vi "IDS Camera Messenger.vi"(0 "Notifier Name":string, 2 "IDS Actions":T5, 5 "IDS Parameter":T1, 7 "ROI Setup":T3, 9 "# of Frames":u32, 11 "File Save Path":path) -> (4 "Notifier Name (Dup)":string, 6 "IDS Parameter":T1, 8 "IDS ROI":T3, 10 "Running?":bool, 13 "Image Ref":T4, 15 "Error?":bool)   [LabVIEW 2025]
uses:
  IDS Controls/IDS Actions.ctl
  IDS Controls/IDS Parameters.ctl
  IDS Controls/IDS Parameter List.ctl
  IDS Controls/IDS ROI.ctl
  <vilib>/vision/Image Controls.llb/IMAQ Image.ctl
  IDS Controls/IDS Notifier Element.ctl
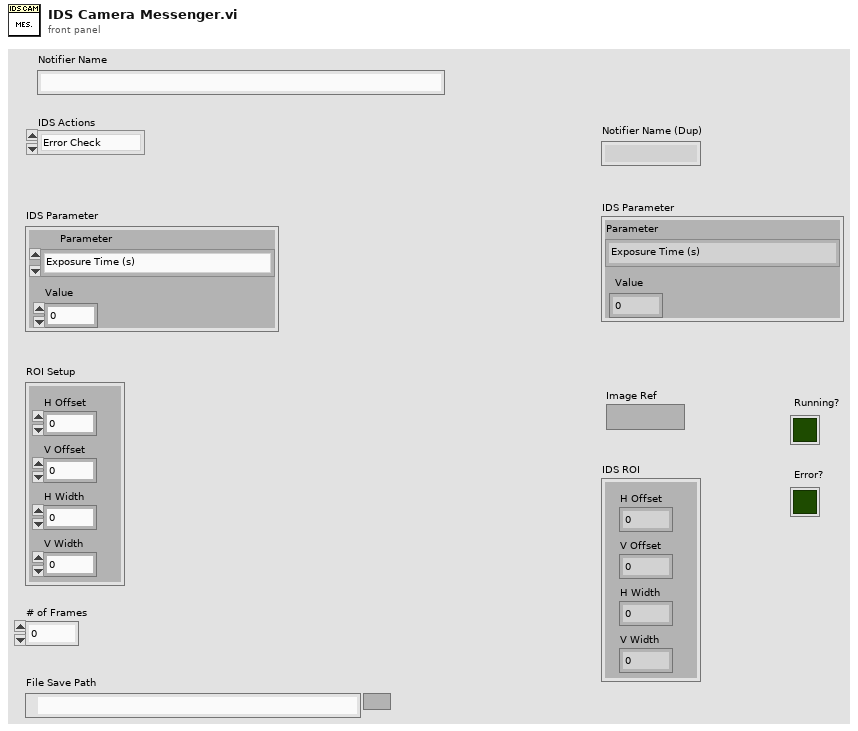
[diagram p1: front panel]
types:
  T1 = typedef "IDS Parameters.ctl" = cluster{"Parameter":T2, "Value":dbl}
  T2 = typedef "IDS Parameter List.ctl" = enum16{"Exposure Time (s)", "Binning"}
  T3 = typedef "IDS ROI.ctl" = cluster{"H Offset":i32, "V Offset":i32, "H Width":i32, "V Width":i32}
  T4 = typedef "IMAQ Image.ctl" = refnum<image>
  T5 = typedef "IDS Actions.ctl" = enum16{"Error Check", "Initialize", "Preview", "Record", "Abort", "Record Settings", "Set Parameter", "Get Parameter", "Set ROI", "Get ROI", "Status", "Quit"}
  T6 = typedef "IDS Notifier Element.ctl" = cluster{"IDS Actions":T5, "Received?":bool, "IDS Parameter":T1, "IDS ROI":T3, "Running?":bool, "File Path":path, "# of frames":u32, "Image Ref":T4, "Error":errorcluster, "Binning":i32}
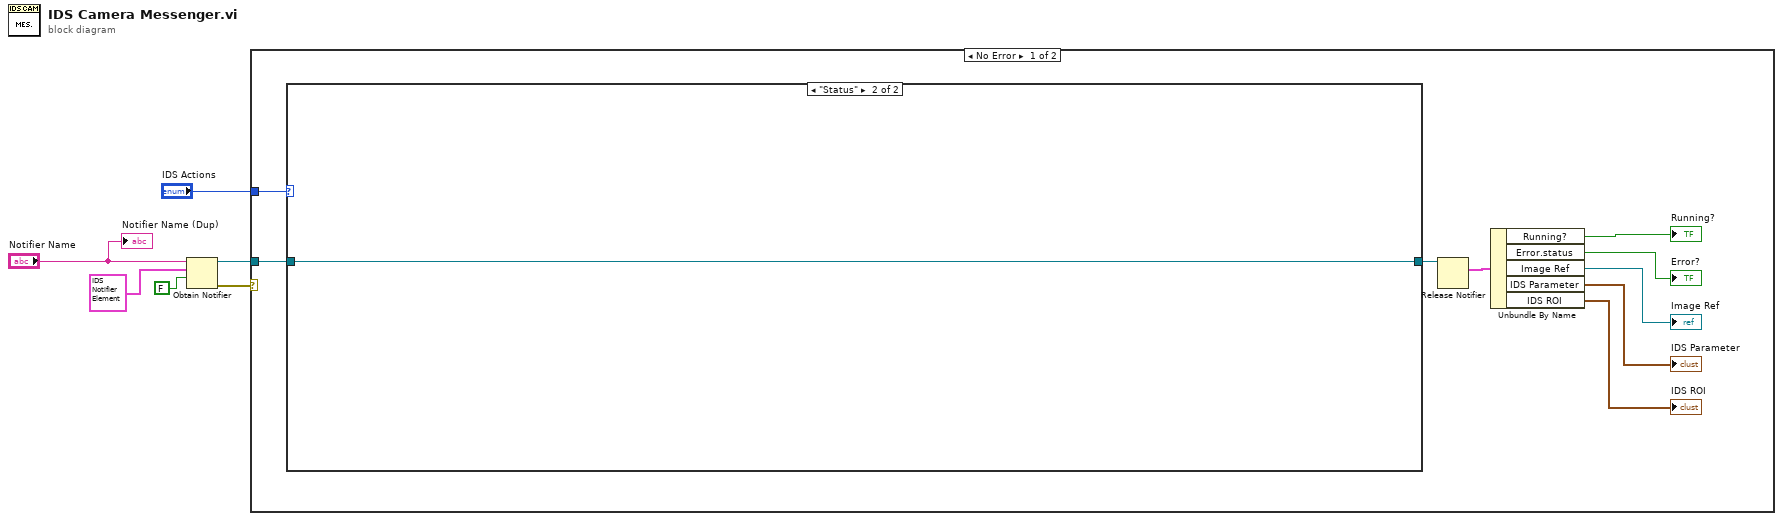
[diagram p0: block diagram]
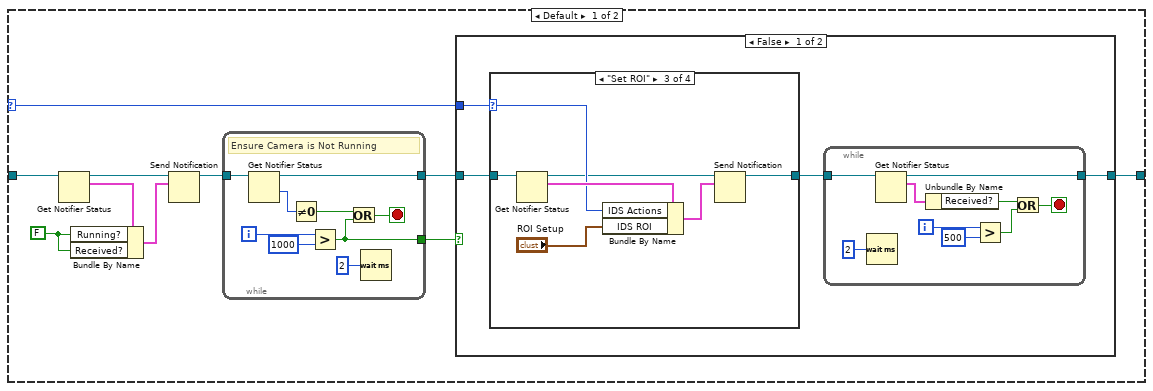
[diagram p2: hidden frame]
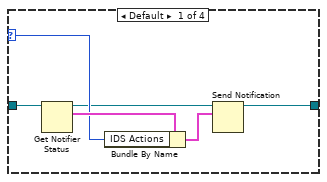
[diagram p3: hidden frame]
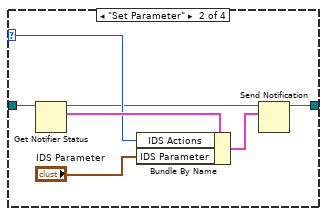
[diagram p4: hidden frame]
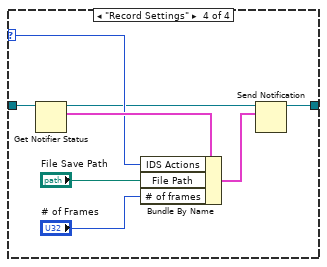
[diagram p5: hidden frame]
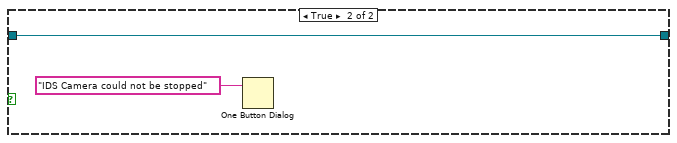
[diagram p6: hidden frame]
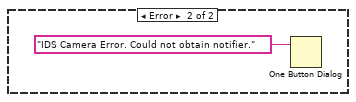
[diagram p7: hidden frame]
diagram:
  n1 = Obtain Notifier(name (unnamed)="Notifier Name", notification data type=T6 {"IDS Actions"=enum."Quit", "Received?"=TRUE, "IDS Parameter"={"Parameter"=enum."Exposure Time (s)", "Value"=0.0}, "IDS ROI"={"H Offset"=0, "V Offset"=0, "H Width"=0, "V Width"=0}, "Running?"=FALSE, "File Path"=path "", "# of frames"=0, "Image Ref"=refnum, "Error"={"status"=FALSE, "code"=0, "source"=""}, "Binning"=0} ("IDS Camera Cluster"), create if not found? (T)=FALSE) -> (notifier out=w3:refnum<notifier>, error out=w4:errorcluster)  [unwired: 1 in, 1 out]
  n2 = case shown="No Error" w4 {
    tunnel: w3 -> [w15 _]
    tunnel: "IDS Actions" -> [w14 _]
    frame No Error {
      n3 = case shown="\"Status\"" w14 {
        selector: w14 -> [w21 _]
        tunnel: w15 -> [w25 w78]
        tunnel: [w20 w78] -> w8
        frame Default {
          w16 = FALSE ("Running?")
          n4 = Get Notifier Status(notifier=w25) -> (notifier out=w19:refnum<notifier>, current notification=w18:T6)  [unwired: 1 in, 3 out]
          n5 = Bundle By Name(cluster=w18, "Running?"=w16, "Received?"=w16) -> (w17:T6)
          n6 = Send Notification(notification=w17, notifier=w19) -> (notifier out=w24:refnum<notifier>)  [unwired: 1 in, 1 out]
          n7 = while {
            tunnel: w24 -> [w77]
            tunnel: [w76] -> w22
            tunnel: [w71] -> w23
            i -> [w73]
            stop <- w75 stop-if-true
            # "Ensure Camera is Not Running"
            n8 = Get Notifier Status(notifier=w77) -> (notifier out=w76:refnum<notifier>, # waiting=w70:i32)  [unwired: 1 in, 3 out]
            n9 = Not Equal To 0?(x=w70) -> (x != 0?=w69:bool)
            n10 = Greater?(x=w73, y=1000) -> (0:w71:bool)
            n11 = Or(x=w69, y=w71) -> (x .or. y?=w75:bool)
            n12 = Wait (ms)(milliseconds to wait=u32 2) -> ()  [unwired: 1 out]
          }
          n13 = case shown="False" w23 {
            tunnel: w22 -> [w27 w67]
            tunnel: w21 -> [w29 _]
            tunnel: [w26 w67] -> w20
            frame False {
              n14 = case shown="\"Set ROI\"" w29 {
                selector: w29 -> [w42 w49 w56 w64]
                tunnel: w27 -> [w44 w51 w58 w66]
                tunnel: [w39 w46 w53 w61] -> w28
                frame Default {
                  n15 = Get Notifier Status(notifier=w44) -> (notifier out=w41:refnum<notifier>, current notification=w43:T6)  [unwired: 1 in, 3 out]
                  n16 = Bundle By Name(cluster=w43, "IDS Actions"=w42) -> (w40:T6)
                  n17 = Send Notification(notification=w40, notifier=w41) -> (notifier out=w39:refnum<notifier>)  [unwired: 1 in, 1 out]
                }
                frame "Set Parameter" {
                  n18 = Get Notifier Status(notifier=w51) -> (notifier out=w48:refnum<notifier>, current notification=w50:T6)  [unwired: 1 in, 3 out]
                  n19 = Bundle By Name(cluster=w50, "IDS Actions"=w49, "IDS Parameter"="IDS Parameter") -> (w47:T6)
                  n20 = Send Notification(notification=w47, notifier=w48) -> (notifier out=w46:refnum<notifier>)  [unwired: 1 in, 1 out]
                }
                frame "Set ROI" {
                  n21 = Get Notifier Status(notifier=w58) -> (notifier out=w55:refnum<notifier>, current notification=w57:T6)  [unwired: 1 in, 3 out]
                  n22 = Bundle By Name(cluster=w57, "IDS Actions"=w56, "IDS ROI"="ROI Setup") -> (w54:T6)
                  n23 = Send Notification(notification=w54, notifier=w55) -> (notifier out=w53:refnum<notifier>)  [unwired: 1 in, 1 out]
                }
                frame "Record Settings" {
                  n24 = Get Notifier Status(notifier=w66) -> (notifier out=w63:refnum<notifier>, current notification=w65:T6)  [unwired: 1 in, 3 out]
                  n25 = Bundle By Name(cluster=w65, "IDS Actions"=w64, "File Path"="File Save Path", "# of frames"="# of Frames") -> (w62:T6)
                  n26 = Send Notification(notification=w62, notifier=w63) -> (notifier out=w61:refnum<notifier>)  [unwired: 1 in, 1 out]
                }
              }
              n27 = while {
                tunnel: w28 -> [w38]
                tunnel: [w30] -> w26
                i -> [w35]
                stop <- w31 stop-if-true
                n28 = Wait (ms)(milliseconds to wait=u32 2) -> ()  [unwired: 1 out]
                n29 = Get Notifier Status(notifier=w38) -> (notifier out=w30:refnum<notifier>, current notification=w37:T6)  [unwired: 1 in, 3 out]
                n30 = Unbundle By Name(w37) -> ("Received?"=w36:bool)
                n31 = Greater?(x=w35, y=500) -> (0:w33:bool)
                n32 = Or(x=w36, y=w33) -> (x .or. y?=w31:bool)
              }
            }
            frame True {
              n33 = One Button Dialog(message="IDS Camera could not be stopped") -> ()  [unwired: 1 in, 1 out]
            }
          }
        }
        frame "Status" {
        }
      }
      n34 = Release Notifier(notifier=w8) -> (last notification=w7:T6)  [unwired: 2 in, 2 out]
      n35 = Unbundle By Name(w7) -> ("Running?"=→"Running?":bool, "Error.status"=→"Error?":bool, "Image Ref"=→"Image Ref":T4, "IDS Parameter"=→"IDS Parameter":T1, "IDS ROI"=→"IDS ROI":T3)
    }
    frame Error {
      n36 = One Button Dialog(message="IDS Camera Error. Could not obtain notifier.") -> ()  [unwired: 1 in, 1 out]
    }
  }
  "Notifier Name (Dup)" <- "Notifier Name"
